vi "Extract Circle Information.vi"(0 "Circle Data":T1(array[cluster])) -> (1 "Circle bounding rectangle":cluster{i32, i32, i32, i32}, 2 "Circle x and y":cluster{"Pos. X":i32, "Pos. Y":i32})   [LabVIEW 2010]
panel:
  # "Circle 1 info"
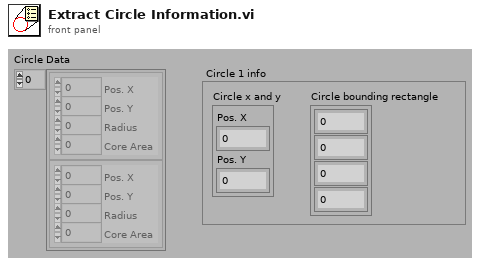
[diagram p1: front panel]
types:
  T1 = cluster{"Pos. X":i32, "Pos. Y":i32, "Radius":i32, "Core Area":i32}[]
  T2 = cluster{"Pos. X":i32, "Pos. Y":i32, "Radius":i32, "Core Area":i32}
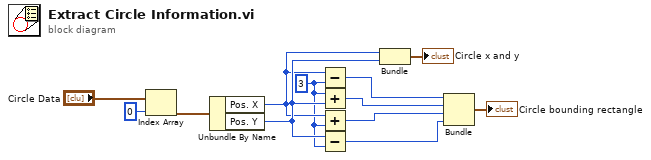
[diagram p0: block diagram]
diagram:
  w5 = 3 ("y")
  n1 = Index Array(array="Circle Data", index=0) -> (element=w6:T2)
  n2 = Unbundle By Name(w6) -> ("Pos. X"=w11:i32, "Pos. Y"=w12:i32)
  n3 = Subtract(x=w11, y=w5) -> (x-y=w7:i32)
  n4 = Add(x=w5, y=w12) -> (x+y=w8:i32)
  n5 = Add(x=w11, y=w5) -> (x+y=w9:i32)
  n6 = Subtract(x=w12, y=w5) -> (x-y=w10:i32)
  n7 = Bundle("Pos. X"=w11, "Pos. Y"=w12) -> (→"Circle x and y":cluster{"Pos. X":i32, "Pos. Y":i32})  [unwired: 1 in]
  n8 = Bundle(w7, w8, w9, w10) -> (→"Circle bounding rectangle":cluster{i32, i32, i32, i32})  [unwired: 1 in]
